vi "Initalize with Switch Parameters.vi"(8 "error in (no error)":errorcluster, 10 "Switch Parameters in":refnum<class "Abstract Switch Init Parameters.lvclass">, 11 "SLSC Switch Consumer in":refnum<class "SLSC Switch Consumer.lvclass">) -> (0 "error out":errorcluster, 3 "SLSC Switch Consumer out":refnum<class "SLSC Switch Consumer.lvclass">)   [LabVIEW 2017, in "SLSC Switch Consumer.lvclass"]
uses:
  SLSC Switch Consumer.lvclass
  Switch/Abstract Switch Init Parameters/Abstract Switch Init Parameters.lvclass
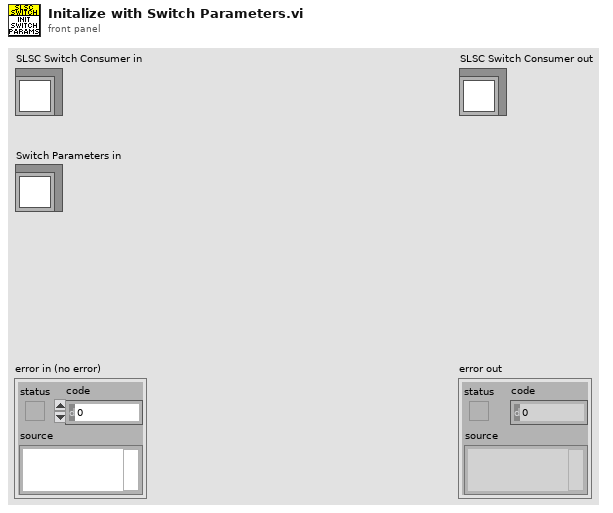
[diagram p1: front panel]
types:
  T1 = typedef "nislscslSession.ctl" = refnum<k20>
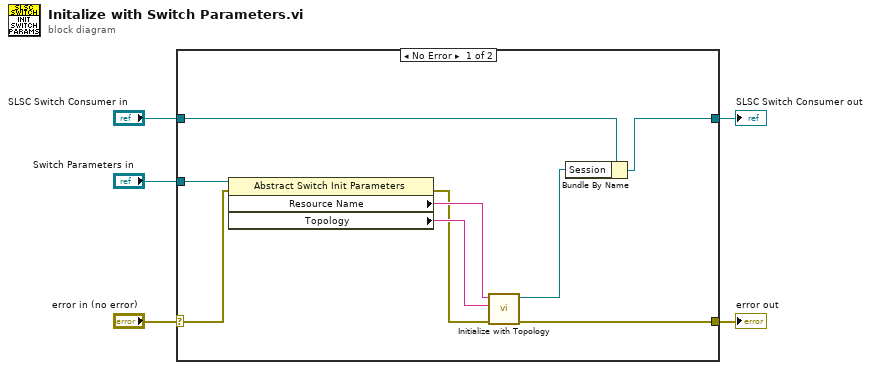
[diagram p0: block diagram]
diagram:
  n1 = case shown="No Error" "error in (no error)" {
    selector: "error in (no error)" -> [w7 w16]
    tunnel: [w9 w16] -> w4
    tunnel: [w12 w15] -> w3
    tunnel: "SLSC Switch Consumer in" -> [w13 w15]
    tunnel: "Switch Parameters in" -> [w14 _]
    frame No Error {
      n2 = property class="Abstract Switch Init Parameters"(reference=w14, error in=w7) -> (error out=w6:errorcluster, "Resource Name"=w11:string, "Topology"=w10:string)  [unwired: 1 out]
      n3 = call <vilib>:"Initialize with Topology.vi"("error in (no error)"=w6, "topology"=w10, "device"=w11) -> ("error out"=w9:errorcluster, "session out"=w8:T1)  [unwired: 7 in]
      n4 = Bundle By Name(cluster=w13, "Session"=w8) -> (w12:refnum<class "SLSC Switch Consumer.lvclass">)
    }
    frame Error {
    }
  }
  "error out" <- w4
  "SLSC Switch Consumer out" <- w3
